vi "Create GB (old).vi"(6 "Edge Duplication Range":dbl=3.0, 7 "Skip crop if no subset":bool, 8 "Reduce to Repeating":T1={"Slab X"=4.6, "Slab Y"=4.0, "Tolerance (A)"=0.5, "Presorted?"=FALSE}, 9 "Min Seperation Distance (A)":dbl=1.5, 10 "Grain Growth and Geometry":T2={"Grain 1 Length (A)"=23.0, "Grain 2 Length (A)"=23.0, "Max Grain Height"=80.0, "Max Grain Width"=14.01, "Grain 1 Start"=0.0, "Overlap Region (A)"=0.0}, 11 "Grain Boundary Definition":T3={"Grain 1 Orientation"=[1.0, 1.0, 1.0], "Grain 2 Orientation"=[1.0, 1.0, 1.0], "Twist Angle (Deg)"=60.0, "Translation Vector"=[0.0, 0.0, 0.0]}) -> (0 "Tilt Angle":dbl, 1 "Subset for Y?":bool=TRUE, 2 "Subset for X?":bool, 3 "Grain Boundary":T4={"Structure Name"="CdTe Expanded to Box+CdTe Expanded to Box", "Lattice vector a"=[20.0, 0.0, 0.0], "Lattice vector b"=[0.0, 89.12914368966783, 0.0], "Lattice vector c"=[0.0, 0.0, 23.299999999999997], "Atoms Array"=[{"Atom Name"="Cd", "Positions (Direct)"=[], "Positions (Cartesian)"=[]}, {"Atom Name"="Te", "Positions (Direct)"=[], "Positions (Cartesian)"=[]}], "# of atoms"=1312} {"Atoms Array"."Positions (Cartesian)" format="%#_4f"; "Atoms Array"."Positions (Direct)" format="%#_4f"})   [LabVIEW 2010]
uses:
  <vilib>/Analysis/_algsub.llb/Real Vector Norm.vi
  <vilib>/Analysis/baseanly.llb/Real A x B.vi
  <vilib>/Analysis/baseanly.llb/Real Dot Product.vi
  <vilib>/Analysis/NI_AALBase.lvlib
  <vilib>/Analysis/NI_AALPro.lvlib
panel:
  out "Time to Crop":u32
  out "Time to find subset":u32
  out "Time to Grow to Box":u32
  out "Time to create primitives":u32
  out "# of Atoms Removed":i32=71
  out "Repeating Y Length Scale":dbl=89.12914368966783
  out "Repeating X Length Scale":dbl
  out "Mutual Viewing Angle":dbl[](array[numeric])=[1.0, -1.0, 0.0]
  in  "Conventional Unit Cell":T4={"Structure Name"="CdTe", "Lattice vector a"=[6.615785553057252, 0.0, 0.0], "Lattice vector b"=[0.0, 6.615785553057252, 0.0], "Lattice vector c"=[0.0, 0.0, 6.615785553057252], "Atoms Array"=[{"Atom Name"="Cd", "Positions (Direct)"=[[0.0, 0.0, 0.0], [0.0, 0.5, 0.5], [0.5, 0.0, 0.5], [0.5, 0.5, 0.0]], "Positions (Cartesian)"=[[0.0, 0.0, 0.0], [0.0, 3.307892776528626, 3.307892776528626], [3.307892776528626, 0.0, 3.307892776528626], [3.307892776528626, 3.307892776528626, 0.0]]}, {"Atom Name"="Te", "Positions (Direct)"=[[0.25, 0.25, 0.25], [0.75, 0.75, 0.25], [0.75, 0.25, 0.75], [0.25, 0.75, 0.75]], "Positions (Cartesian)"=[[1.653946388264313, 1.653946388264313, 1.653946388264313], [4.96183916479294, 4.96183916479294, 1.653946388264313], [4.96183916479294, 1.653946388264313, 4.96183916479294], [1.653946388264313, 4.96183916479294, 4.96183916479294]]}], "# of atoms"=8}
  # "Primitives"
  # "Grain Growth"
  # "Remove Collisions"
  # "Make into repeating cell"
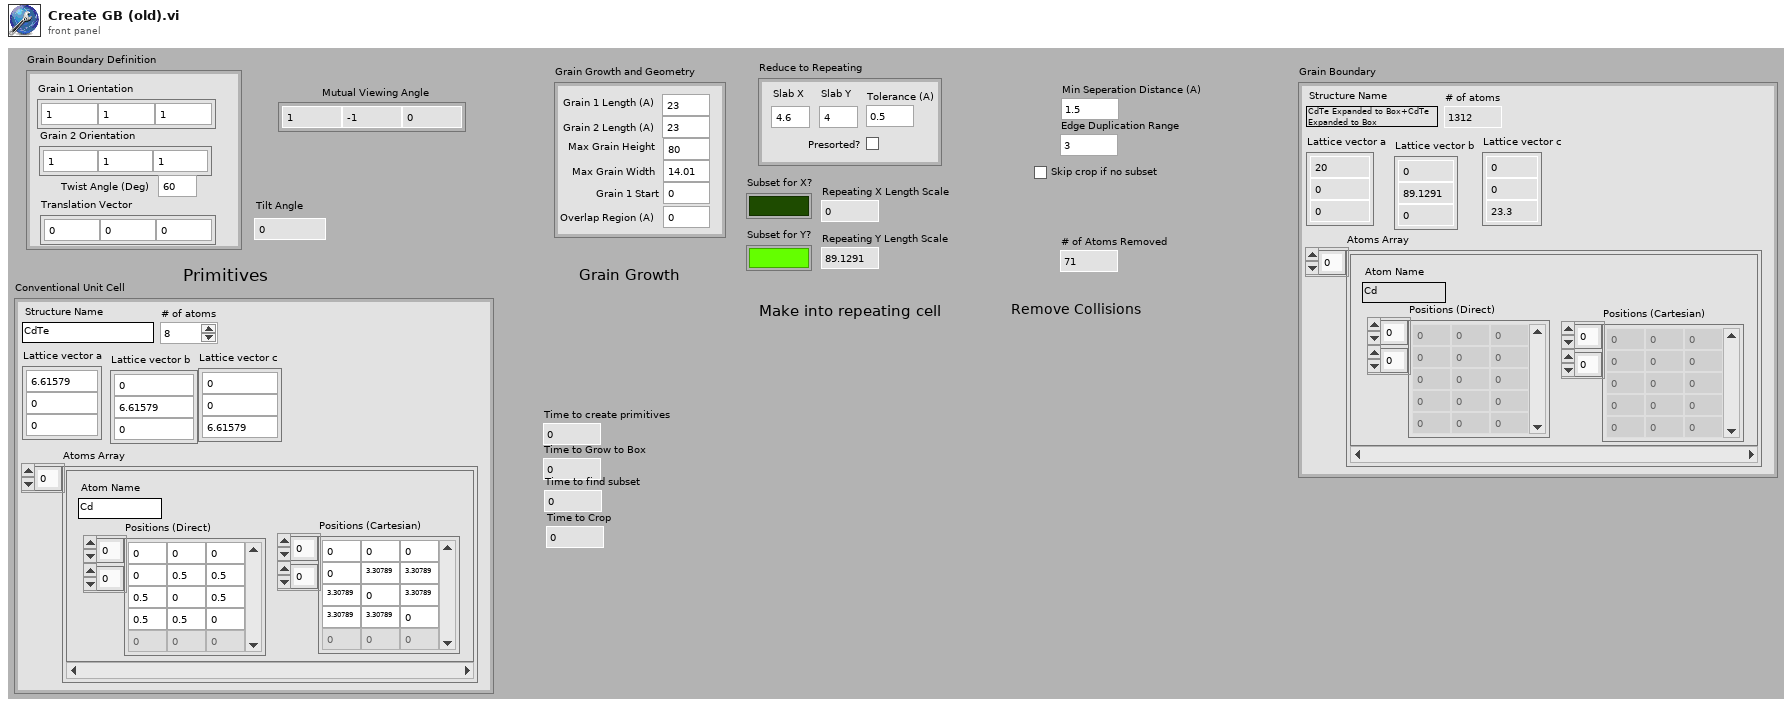
[diagram p1: front panel]
types:
  T1 = cluster{"Slab X":dbl, "Slab Y":dbl, "Tolerance (A)":dbl, "Presorted?":bool}
  T2 = cluster{"Grain 1 Length (A)":dbl, "Grain 2 Length (A)":dbl, "Max Grain Height":dbl, "Max Grain Width":dbl, "Grain 1 Start":dbl, "Overlap Region (A)":dbl}
  T3 = cluster{"Grain 1 Orientation":dbl[], "Grain 2 Orientation":dbl[], "Twist Angle (Deg)":dbl, "Translation Vector":dbl[]}
  T4 = cluster{"Structure Name":string, "Lattice vector a":dbl[], "Lattice vector b":dbl[], "Lattice vector c":dbl[], "Atoms Array":cluster{"Atom Name":string, "Positions (Direct)":dbl[][], "Positions (Cartesian)":dbl[][]}[], "# of atoms":i32}
  T5 = typedef "NI_Matrix.lvlib/RealMatrix.ctl" = dbl[][]
  T6 = cluster{"Z Min":dbl, "Max Grain Width":dbl, "Z Min":dbl, "Max Grain Height":dbl, "Grain 1 Start":dbl, "Grain 1 Length (A)":dbl}
  T7 = cluster{"Grain 1 Start":dbl, "Max Grain Width":dbl, "Grain 1 Start":dbl, "Max Grain Height":dbl, dbl, "Grain 2 Length (A)":dbl}
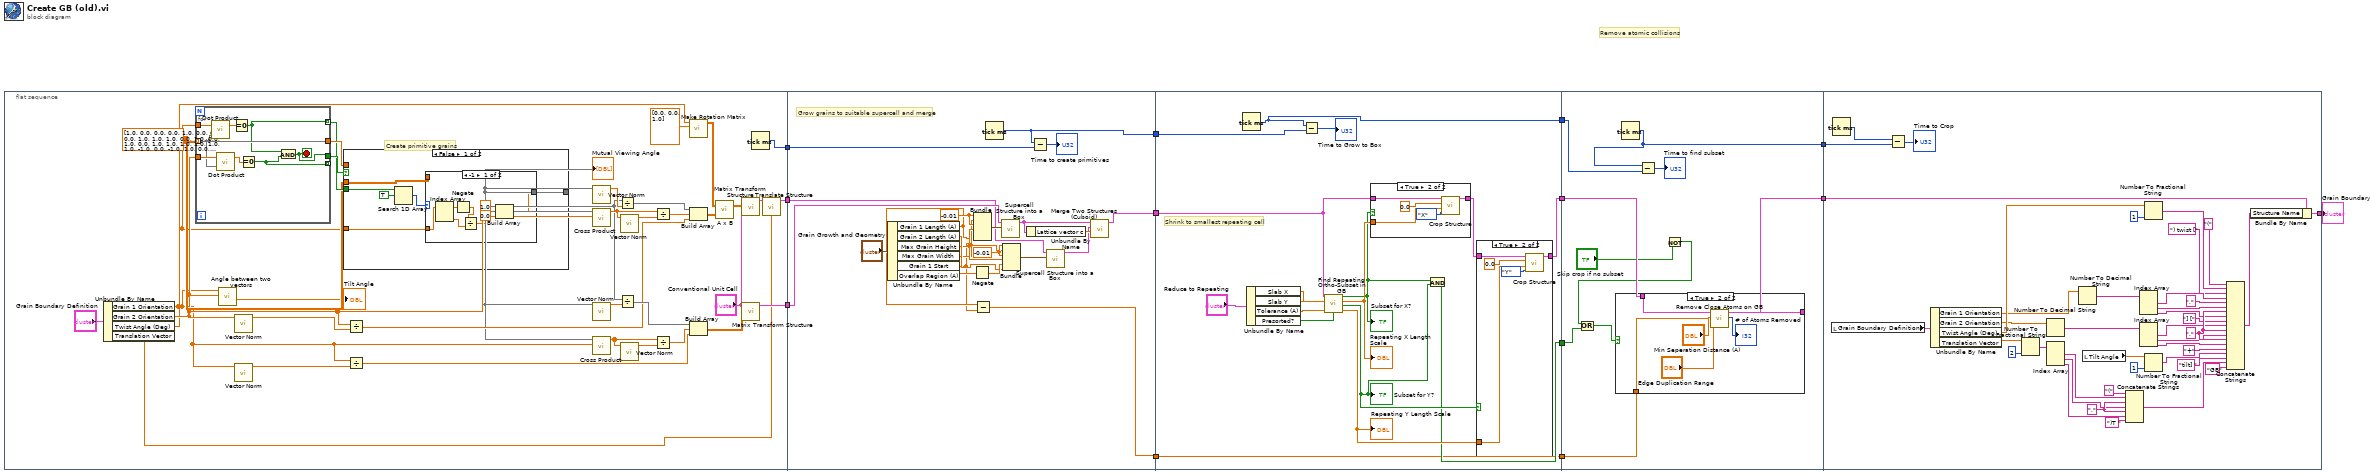
[diagram p0: block diagram]
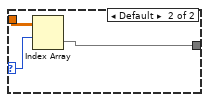
[diagram p2: hidden frame]
diagram:
  # "Remove atomic collisions"
  n1 = flat-sequence {
    tunnel: [w22] -> w13
    tunnel: [w36] -> w12
    tunnel: [w14] -> w6
    tunnel: w13 -> [w90]
    tunnel: w12 -> [w94]
    tunnel: [w86] -> w8
    tunnel: w6 -> [w79]
    tunnel: [w78] -> w5
    tunnel: [w75] -> w2
    tunnel: w8 -> [w110]
    tunnel: [w109] -> w10
    tunnel: [w101] -> w7
    tunnel: w5 -> [w100]
    tunnel: [w98] -> w4
    tunnel: w2 -> [w97]
    tunnel: [w97] -> w1
    tunnel: w10 -> [w135]
    tunnel: [w134] -> w9
    tunnel: w7 -> [w130]
    tunnel: w4 -> [w132]
    tunnel: [w131] -> w3
    tunnel: w1 -> [w126]
    tunnel: [w146] -> w11
    tunnel: w9 -> [w148]
    tunnel: w3 -> [w143]
    frame #0 {
      w45 = dbl[][] [[1.0, 0.0, 0.0], [0.0, 1.0, 0.0], [0.0, 0.0, 1.0], [1.0, 1.0, 0.0], [1.0, 0.0, 1.0], [0.0, 1.0, 1.0], [1.0, 1.0, 1.0], [1.0, -1.0, 0.0], [-1.0, 1.0, 0.0], [1.0, 0.0, -1.0], [-1.0, 0.0, 1.0], [0.0, -1.0, 1.0], [0.0, 1.0, -1.0], [1.0, -1.0, 1.0], [-1.0, 1.0, 1.0], [1.0, 1.0, -1.0]] ("Grain 1 Orientation 2")
      # "Create primitive grains"
      n2 = Unbundle By Name("Grain Boundary Definition") -> ("Grain 1 Orientation"=w15:dbl[], "Grain 2 Orientation"=w18:dbl[], "Twist Angle (Deg)"=w17:dbl, "Translation Vector"=w16:dbl[])
      n3 = for {
        tunnel: w15 -> [w74]
        tunnel: w45 -> [w71] mode=indexing
        tunnel: [w71] -> w47
        tunnel: w18 -> [w72]
        tunnel: [w69] -> w46 mode=indexing
        tunnel: [w68] -> _ mode=indexing
        tunnel: [w67] -> w48
        stop <- w67 stop-if-true
        n4 = call-poly <vilib>:"Dot Product.vi"("Y Vector"=w71, "X Vector"=w74) -> ("X * Y"=w73:dbl)  [unwired: 1 out]
        n5 = call-poly <vilib>:"Dot Product.vi"("Y Vector"=w71, "X Vector"=w72) -> ("X * Y"=w70:dbl)  [unwired: 1 out]
        n6 = Equal To 0?(x=w73) -> (x = 0?=w69:bool)
        n7 = Equal To 0?(x=w70) -> (x = 0?=w68:bool)
        n8 = And(x=w69, y=w68) -> (x .and. y?=w67:bool)
      }
      n9 = call "Angle between two vectors.vi"("Vector 2"=w18, "Vector 1"=w15) -> ("Angle (Degrees)"=→"Tilt Angle":dbl)  [unwired: 7 in, 2 out]
      n10 = call-poly <vilib>:"Vector Norm.vi"("Input Vector"=w18) -> ("norm"=w26:dbl)  [unwired: 9 in, 1 out]
      n11 = call-poly <vilib>:"Vector Norm.vi"("Input Vector"=w15) -> ("norm"=w42:dbl)  [unwired: 9 in, 1 out]
      n12 = case shown="False" w48 {
        tunnel: w47 -> [_ w66]
        tunnel: [w51 w66] -> w23
        tunnel: w46 -> [w54 _]
        tunnel: w45 -> [w52 _]
        tunnel: w15 -> [w49 _]
        frame False {
          n13 = Search 1D Array(1D array=w54, element=TRUE) -> (index of element=w50:i32)  [unwired: 1 in]
          n14 = case shown="-1" w50 {
            selector: w50 -> [_ w63]
            tunnel: w52 -> [_ w65]
            tunnel: [w55 w64] -> w51
            tunnel: w49 -> [w60 _]
            frame -1 {
              n15 = Index Array(array=w60) -> (element #1=w59:dbl, element #2=w57:dbl)  [unwired: 2 in]
              n16 = Negate(x=w59) -> (-x=w58:dbl)
              n17 = Divide(x=w58, y=w57) -> (x/y=w56:dbl)
              n18 = Build Array(1.0 ("element"), w56, 0.0 ("element")) -> (w55:dbl[])
            }
            frame Default {
              n19 = Index Array(array=w65, index (row)=w63) -> (element=w64:dbl[])  [unwired: 1 in]
            }
          }
        }
        frame True {
        }
      }
      "Mutual Viewing Angle" <- w23
      n20 = Divide(x=w18, y=w26) -> (x/y=w28:dbl[])
      n21 = Divide(x=w15, y=w42) -> (x/y=w40:dbl[])
      n22 = call-poly <vilib>:"Vector Norm.vi"("Input Vector"=w23) -> ("norm"=w24:dbl)  [unwired: 9 in, 1 out]
      n23 = call <vilib>:"Cross Product.vi"("B Vector"=w18, "A Vector"=w23) -> ("Cross Product"=w29:dbl[])  [unwired: 8 in, 1 out]
      n24 = call-poly <vilib>:"Vector Norm.vi"("Input Vector"=w23) -> ("norm"=w44:dbl)  [unwired: 9 in, 1 out]
      n25 = call <vilib>:"Cross Product.vi"("B Vector"=w15, "A Vector"=w23) -> ("Cross Product"=w38:dbl[])  [unwired: 8 in, 1 out]
      n26 = Divide(x=w23, y=w24) -> (x/y=w27:dbl[])
      n27 = Divide(x=w23, y=w44) -> (x/y=w41:dbl[])
      n28 = call-poly <vilib>:"Vector Norm.vi"("Input Vector"=w29) -> ("norm"=w25:dbl)  [unwired: 9 in, 1 out]
      n29 = call-poly <vilib>:"Vector Norm.vi"("Input Vector"=w38) -> ("norm"=w43:dbl)  [unwired: 9 in, 1 out]
      n30 = Divide(x=w29, y=w25) -> (x/y=w35:dbl[])
      n31 = Divide(x=w38, y=w43) -> (x/y=w37:dbl[])
      n32 = call "Make Rotation Matrix.vi"("Rotation Axis"=dbl[] [0.0, 0.0, 1.0], "Rotation Angle (Degree)"=w17) -> ("Rotation Matrix"=w32:T5)  [unwired: 9 in]
      n33 = Build Array(w27, w35, w28) -> (w33:T5)
      n34 = Build Array(w41, w37, w40) -> (w39:T5)
      n35 = call-poly <vilib>:"A x B.vi"("B"=w33, "A"=w32) -> ("A x B"=w31:T5)  [unwired: 1 out]
      n36 = call "Matrix Transform Structure.vi"("Matrix Transform"=w31, "Original Structure"="Conventional Unit Cell") -> ("After Transform"=w34:T4)  [unwired: 9 in]
      n37 = call "Matrix Transform Structure.vi"("Matrix Transform"=w39, "Original Structure"="Conventional Unit Cell") -> ("After Transform"=w36:T4)  [unwired: 9 in]
      n38 = Tick Count (ms)() -> (millisecond timer value=w14:u32)
      n39 = call "Translate Structure.vi"("Translation Vector (Cartesian)"=w16, "Atomic Structure"=w34) -> ("Shifted Structure"=w22:T4)  [unwired: 9 in]
    }
    frame #1 {
      w93 = -0.01 ("Z Min")
      w96 = -0.01 ("Grain 1 Start")
      # "Grow grains to suitable supercell and merge"
      n40 = Unbundle By Name("Grain Growth and Geometry") -> ("Grain 1 Length (A)"=w77:dbl, "Grain 2 Length (A)"=w84:dbl, "Max Grain Height"=w82:dbl, "Max Grain Width"=w81:dbl, "Grain 1 Start"=w76:dbl, "Overlap Region (A)"=w83:dbl)
      n41 = Negate(x=w83) -> (-x=w95:dbl)
      n42 = Bundle("Z Min"=w93, "Max Grain Width"=w81, "Z Min"=w93, "Max Grain Height"=w82, "Grain 1 Start"=w76, "Grain 1 Length (A)"=w77) -> (w92:T6)  [unwired: 1 in]
      n43 = Subtract(x=w77, y=w76) -> (x-y=w75:dbl)
      n44 = Tick Count (ms)() -> (millisecond timer value=w78:u32)
      n45 = call "Supercell Structure into a Box.vi"("Draw Box"=w92, "Subcrystal"=w94) -> ("Expanded cubic Structure"=w87:T4)  [unwired: 7 in, 2 out]
      n46 = Bundle("Grain 1 Start"=w96, "Max Grain Width"=w81, "Grain 1 Start"=w96, "Max Grain Height"=w82, w95, "Grain 2 Length (A)"=w84) -> (w91:T7)  [unwired: 1 in]
      n47 = Unbundle By Name(w87) -> ("Lattice vector c"=w89:dbl[])
      n48 = Subtract(x=w78, y=w79) -> (x-y=→"Time to create primitives":u32)
      n49 = call "Supercell Structure into a Box.vi"("Draw Box"=w91, "Subcrystal"=w90) -> ("Expanded cubic Structure"=w88:T4)  [unwired: 7 in, 2 out]
      n50 = call "Merge Two Structures (Cuboid).vi"("Translation Vector (1 to 2)"=w89, "Atomic Structure 2"=w88, "Atomic Structure 1"=w87) -> ("Atomic Structure of 1 + 2 by T"=w86:T4)  [unwired: 8 in]
    }
    frame #2 {
      # "Shrink to smallest repeating cell"
      n51 = Tick Count (ms)() -> (millisecond timer value=w98:u32)
      n52 = Unbundle By Name("Reduce to Repeating") -> ("Slab X"=w107:dbl, "Slab Y"=w106:dbl, "Tolerance (A)"=w105:dbl, "Presorted?"=w104:bool)
      n53 = Subtract(x=w98, y=w100) -> (x-y=→"Time to Grow to Box":u32)
      n54 = call "Find Repeating Ortho-Subset in GB.vi"("Presorted?"=w104, "Tolerance (A)"=w105, "Slab Y"=w106, "Slab X"=w107, "Grain Boundary"=w110) -> ("Repeating Y Length Scale"=w111:dbl, "Subset Y found?!"=w102:bool, "Repeating X Length Scale"=w112:dbl, "Subset X found?!"=w103:bool)  [unwired: 3 in]
      "Repeating X Length Scale" <- w112
      "Subset for X?" <- w103
      "Repeating Y Length Scale" <- w111
      "Subset for Y?" <- w102
      n55 = case shown="True" w103 {
        tunnel: w110 -> [w120 w125]
        tunnel: [w120 w122] -> w113
        tunnel: w112 -> [_ w121]
        frame False {
        }
        frame True {
          n56 = call "Crop Structure.vi"("Cropping Index"=enum16{"X", "Y", "Z"}."X", "Upper Bound Z"=w121, "Lower bound Z"=0.0, "Input Structure"=w125) -> ("Cropped Structure"=w122:T4)  [unwired: 7 in]
        }
      }
      n57 = And(x=w103, y=w102) -> (x .and. y?=w101:bool)
      n58 = case shown="True" w102 {
        tunnel: w113 -> [w114 w119]
        tunnel: w111 -> [_ w117]
        tunnel: [w114 w115] -> w109
        frame False {
        }
        frame True {
          n59 = call "Crop Structure.vi"("Cropping Index"=enum16{"X", "Y", "Z"}."Y", "Upper Bound Z"=w117, "Lower bound Z"=0.0, "Input Structure"=w119) -> ("Cropped Structure"=w115:T4)  [unwired: 7 in]
        }
      }
    }
    frame #3 {
      n60 = Tick Count (ms)() -> (millisecond timer value=w131:u32)
      n61 = Subtract(x=w131, y=w132) -> (x-y=→"Time to find subset":u32)
      n62 = Not(x="Skip crop if no subset") -> (.not. x?=w127:bool)
      n63 = Or(x=w127, y=w130) -> (x .or. y?=w129:bool)
      n64 = case shown="True" w129 {
        tunnel: w135 -> [w136 w140]
        tunnel: [w136 w139] -> w134
        tunnel: w126 -> [_ w137]
        frame False {
        }
        frame True {
          n65 = call "Remove Close Atoms on GB.vi"("Grain Boundary Location (A)"=w137, "Edge Duplication Range"="Edge Duplication Range", "Minimally Allowable Distance (A)"="Min Seperation Distance (A)", "Structure"=w140) -> ("# of Atoms Removed"=→"# of Atoms Removed":i32, "Structure with atoms removed"=w139:T4)  [unwired: 6 in]
        }
      }
    }
    frame #4 {
      w173 = "," ("string")
      w160 = "," ("string")
      n66 = local read "Grain Boundary Definition"() -> (w178:T3)
      n67 = Tick Count (ms)() -> (millisecond timer value=w144:u32)
      n68 = Subtract(x=w144, y=w143) -> (x-y=→"Time to Crop":u32)
      n69 = Unbundle By Name(w178) -> ("Grain 1 Orientation"=w179:dbl[], "Grain 2 Orientation"=w180:dbl[], "Twist Angle (Deg)"=w181:dbl, "Translation Vector"=w182:dbl[])
      n70 = Number To Fractional String(number=w182, precision (6)=i16 2) -> (F-format string=w169:string[])  [unwired: 2 in]
      n71 = Number To Decimal String(number=w180) -> (decimal integer string=w163:string[])  [unwired: 1 in]
      n72 = Index Array(array=w169) -> (element #1=w170:string, element #2=w172:string, element #3=w174:string)  [unwired: 3 in]
      n73 = Number To Decimal String(number=w179) -> (decimal integer string=w162:string[])  [unwired: 1 in]
      n74 = local read "Tilt Angle"() -> (w183:dbl)
      n75 = Concatenate Strings("(" ("string"), w170, w173, w172, w173, w174, ")T " ("string")) -> (w176:string)
      n76 = Index Array(array=w162) -> (element #1=w153:string, element #2=w155:string, element #3=w156:string)  [unwired: 3 in]
      n77 = Index Array(array=w163) -> (element #1=w158:string, element #2=w159:string, element #3=w161:string)  [unwired: 3 in]
      n78 = Number To Fractional String(number=w181, precision (6)=i16 1) -> (F-format string=w151:string)  [unwired: 2 in]
      n79 = Number To Fractional String(number=w183, precision (6)=i16 1) -> (F-format string=w165:string)  [unwired: 2 in]
      n80 = Concatenate Strings("(" ("string"), w151, ") twist [" ("string"), w153, "," ("string"), w155, w160, w156, "] [" ("string"), w158, w160, w159, w160, w161, "+" ("string"), w165, "tilt] " ("string"), w176, "GB" ("string")) -> (w147:string)
      n81 = Bundle By Name(cluster=w148, "Structure Name"=w147) -> (w146:T4)
    }
  }
  "Grain Boundary" <- w11
